vi "Get Image.vi"(8 "error in (no error)":errorcluster, 11 "senseHatDisplay in":refnum<class "RPI.SenseHat.Display.lvclass">) -> (0 "error out":errorcluster, 2 "Image":refnum<class "Image.lvclass">, 3 "senseHatDisplay out":refnum<class "RPI.SenseHat.Display.lvclass">)   [LabVIEW 2020, in "RPI.SenseHat.Display.lvlib" / "RPI.SenseHat.Display.lvclass"]
doc: "Returns the virtual screen array."
uses:
  RPI.SenseHat.Display.lvclass
  Image/Image.lvclass
  RPI.SenseHat.Display.lvclass/RPI.SenseHat.Display.ctl
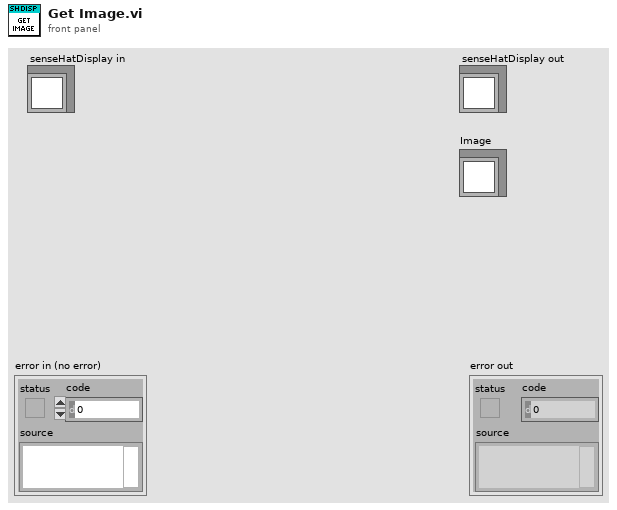
[diagram p1: front panel]
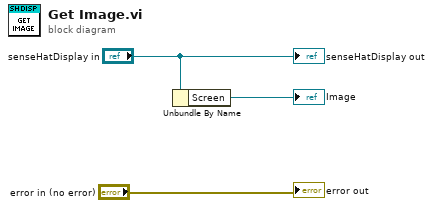
[diagram p0: block diagram]
diagram:
  n1 = Unbundle By Name("senseHatDisplay in") -> ("Screen"=→"Image":refnum<class "Image.lvclass">)
  "error out" <- "error in (no error)"
  "senseHatDisplay out" <- "senseHatDisplay in"
